vi "Ping 1.0.vi"() -> ()   [LabVIEW 2013]
panel:
  out "offset past match":i32
  out "concatenated string":string
  out "IP address":i32
  out "Ping Cout":i32
  in  "file path":path
  out "Array":errorcluster[](array[cluster])
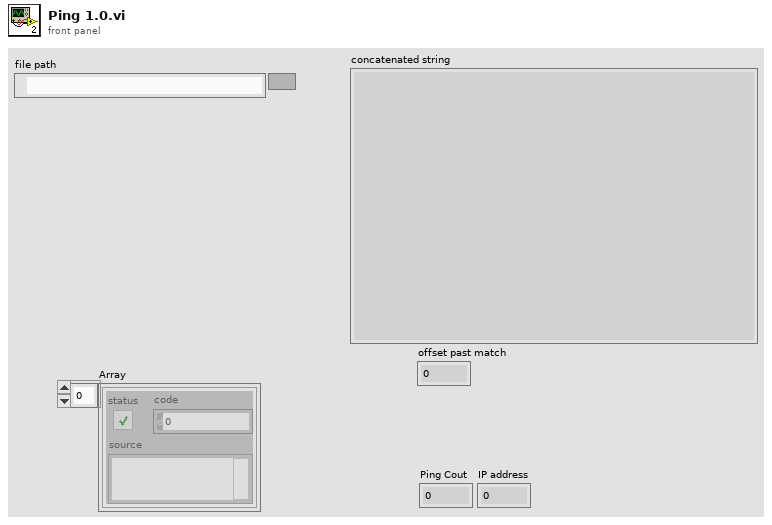
[diagram p1: front panel]
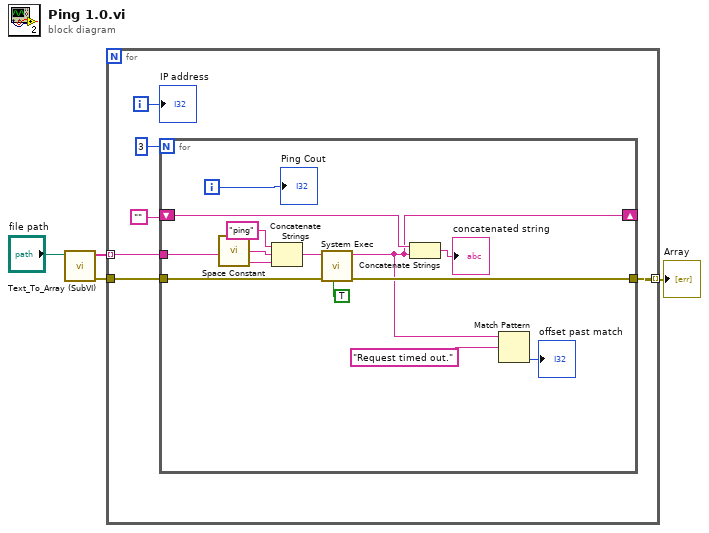
[diagram p0: block diagram]
diagram:
  n1 = call "Text_To_Array (SubVI).vi"("file path"="file path") -> ("error out"=w3:errorcluster, "Array"=w4:string[])  [unwired: 8 in, 1 out]
  n2 = for {
    tunnel: w4 -> [w8] mode=indexing
    tunnel: w3 -> [w10]
    tunnel: [w9] -> w2 mode=indexing
    i -> [w6]
    n3 = for {
      N: 3 -> [_]
      tunnel: w10 -> [w23]
      tunnel: [w22] -> w9
      tunnel: w8 -> [w20]
      shift-right: [w13] -> _
      shift-left: "" -> [w15]
      i -> [w16]
      n4 = call <vilib>:"Space Constant.vi"() -> ("String"=w18:string)
      n5 = Concatenate Strings("ping", w18, w20) -> (w21:string)
      n6 = call <vilib>:"System Exec.vi"("run minimized? (F)"=TRUE, "error in (no error)"=w23, "command line"=w21) -> ("error out"=w22:errorcluster, "standard output"=w13:string)  [unwired: 5 in, 2 out]
      n7 = Concatenate Strings(w15, w13) -> (→"concatenated string":string)
      n8 = Match Pattern(string=w13, regular expression="Request timed out." ("search string/char (-)")) -> (offset past match=→"offset past match":i32)  [unwired: 1 in, 3 out]
      "Ping Cout" <- w16
    }
    "IP address" <- w6
  }
  "Array" <- w2
